vi "Measurement Logic.vi"() -> ()   [LabVIEW 2021, in "Voltage Measurement.lvlib"]
uses:
  Voltage Measurement.lvlib
  Measurement Configuration.ctl
  <instrlib>/niDMM/nidmm.llb/niDMM Resolution in Digits.ctl
  Measurement Results.ctl
  <vilib>/Plug-In SDKs/Measurements/Measure Call Context/Measure Call Context.lvclass
  a4d2c730-40f0-43b4-8942-0e6b76d5927d.vi
  68e02d93-10e8-4ba4-ae91-57667ec1bb5a.vi
  aa39d5ca-b66e-49b6-89c1-6be1f8ef5710.vi
  <vilib>/Plug-In SDKs/Sessions/niDMM/NI Session Management niDMM.lvlib
  <vilib>/Plug-In SDKs/Sessions/niDCPower/NI Session Management niDCPower.lvlib
  <vilib>/Plug-In SDKs/Clients/Session Management V1/Session Reservation/Session Reservation.lvclass
panel:
  out "measure call context out":refnum<class "Measure Call Context.lvclass">
  in  "measure call context in":refnum<class "Measure Call Context.lvclass">
  out "measurement results":T1={"Measurement "=0.0, "Signal Out of Range"=FALSE, "Measurement from SMU Str"="Empty", "Waveform Graph"=[0.0]} {"Measurement" format="%.6p"}
  in  "measurement configuration":T2={"Vin SMU Channel"="Lorem ipsum dolor sit", "Range"=1.2, "Resolution in Digits"=0.0, "Voltage Config Str"="", "Current Config Str"="", "Vin SMU Pin"="", "Device Name Pin"=""} {"Resolution in Digits" items=["3 1/2"=3.5, "4 1/2"=4.5, "5 1/2"=5.5, "6 1/2"=6.5, "7 1/2"=7.5]}
  out "error out":errorcluster
  in  "error in":errorcluster
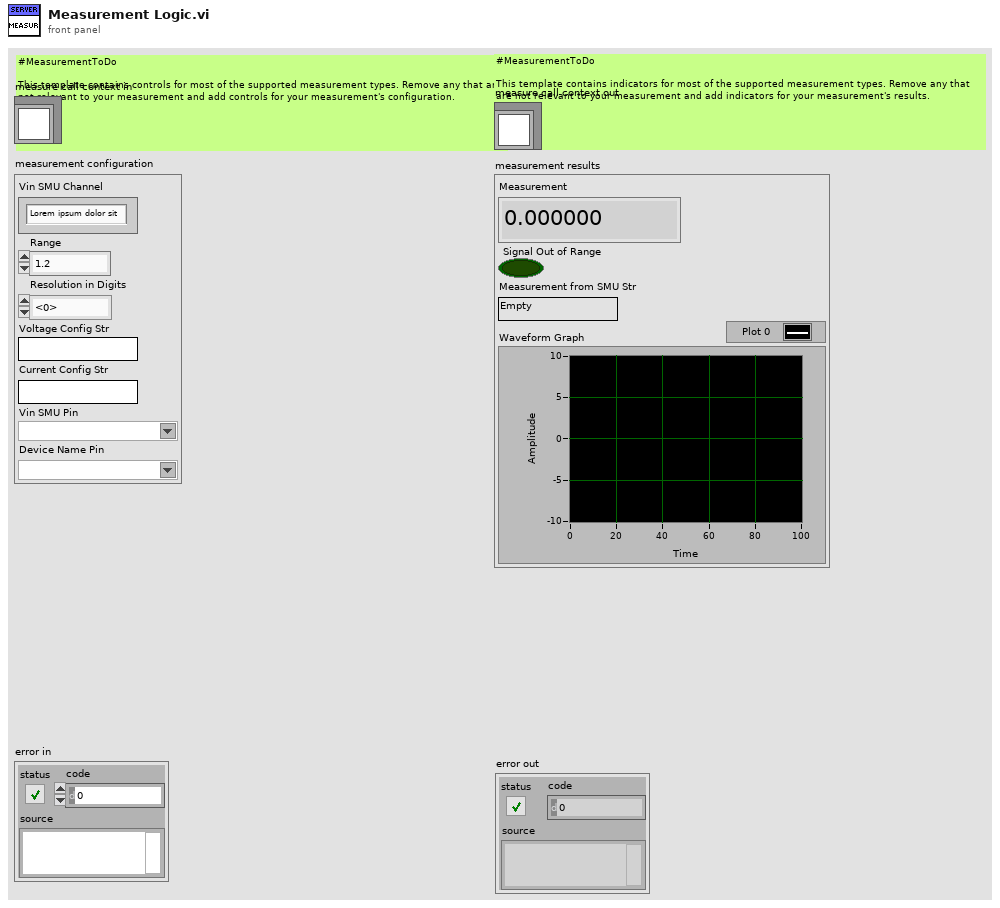
[diagram p1: front panel]
types:
  T1 = typedef "Voltage Measurement.lvlib/Measurement Results.ctl" = cluster{"Measurement ":dbl, "Signal Out of Range":bool, "Measurement from SMU Str":string, "Waveform Graph":dbl[]}
  T2 = typedef "Voltage Measurement.lvlib/Measurement Configuration.ctl" = cluster{"Vin SMU Channel":string, "Range":dbl, "Resolution in Digits":T3, "Voltage Config Str":string, "Current Config Str":string, "Vin SMU Pin":string, "Device Name Pin":string}
  T3 = typedef "niDMM Resolution in Digits.ctl" = dbl
  T4 = typedef "NI Session Management niDMM.lvlib/Connection with Session.ctl" = cluster{"connection":T5, "session":refnum<k15>}
  T5 = typedef "NI Session Management V1 Client.lvlib/Session Reservation.lvclass/Connection.ctl" = cluster{"pin or relay name":string, "site":i32, "instrument type id":string, "channel":string}
  T6 = typedef "NI Session Management niDCPower.lvlib/Connection with Session.ctl" = cluster{"connection":T5, "session":refnum<k15>}
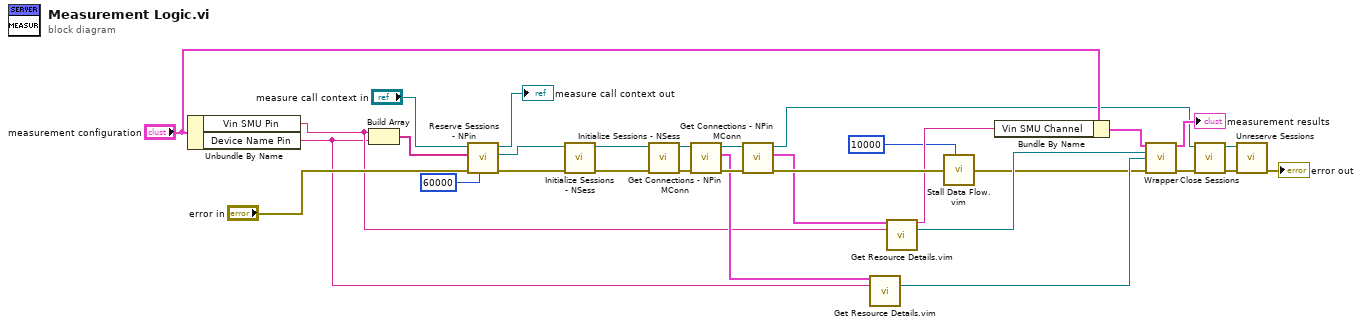
[diagram p0: block diagram]
diagram:
  n1 = Unbundle By Name("measurement configuration") -> ("Vin SMU Pin"=w8:string, "Device Name Pin"=w7:string)
  n2 = Build Array(w8, w7) -> (w27:string[])
  n3 = call <vilib>:"Reserve Sessions - NPin.vi"("timeout (ms)"=60000, "error in"="error in", "pin or relay names"=w27, "measurement context in"="measure call context in") -> ("error out"=w26:errorcluster, "session reservation out"=w25:refnum<class "Session Reservation.lvclass">, "measurement context out"=→"measure call context out":refnum<class "Measure Call Context.lvclass">)  [unwired: 5 in]
  n4 = call <vilib>:"Initialize Sessions - NSess.vi"("error in"=w26, "session reservation in"=w25) -> ("error out"=w24:errorcluster, "session reservation out"=w23:refnum<class "Session Reservation.lvclass">)  [unwired: 6 in, 2 out]
  n5 = call <vilib>:"Initialize Sessions - NSess.vi"("error in"=w24, "session reservation in"=w23) -> ("error out"=w22:errorcluster, "session reservation out"=w21:refnum<class "Session Reservation.lvclass">)  [unwired: 6 in, 2 out]
  n6 = call <vilib>:"Get Connections - NPin MConn.vi"("error in"=w22, "session reservation in"=w21) -> ("error out"=w20:errorcluster, "connections"=w10:T4[], "session reservation out"=w19:refnum<class "Session Reservation.lvclass">)  [unwired: 7 in]
  n7 = call <vilib>:"Get Connections - NPin MConn.vi"("error in"=w20, "session reservation in"=w19) -> ("error out"=w17:errorcluster, "connections"=w9:T6[], "session reservation out"=w15:refnum<class "Session Reservation.lvclass">)  [unwired: 7 in]
  n8 = call "Get Resource Details.vim"("connections"=w10, "Pin Name"=w7) -> ("session"=w4:refnum<k15>)  [unwired: 12 in, 1 out]
  n9 = call "Get Resource Details.vim"("connections"=w9, "Pin Name"=w8) -> ("channel"=w6:string, "session"=w5:refnum<k15>)  [unwired: 12 in]
  n10 = call "Stall Data Flow.vim"("value in"=w17, "milliseconds to wait"=u32 10000) -> ("value out"=w3:errorcluster)  [unwired: 1 out]
  n11 = Bundle By Name(cluster="measurement configuration", "Vin SMU Channel"=w6) -> (w11:T2)
  n12 = call "Wrapper.vi"("measurement configuration"=w11, "Vin SMU"=w5, "Device Name"=w4, "error in"=w3) -> ("measurement results"=→"measurement results":T1, "error out"=w16:errorcluster)  [unwired: 10 in]
  n13 = call <vilib>:"Close Sessions.vi"("error in"=w16, "session reservation in"=w15) -> ("error out"=w13:errorcluster, "session reservation out"=w12:refnum<class "Session Reservation.lvclass">)  [unwired: 8 in]
  n14 = call <vilib>:"Unreserve Sessions.vi"("error in"=w13, "session reservation in"=w12) -> ("error out"=→"error out":errorcluster)  [unwired: 9 in]
